vi "svx_Generate Excitation (DAQmx).vi"(0 "acquisition task":T1={"AI device settings"={"AI DAQmx TaskID"="", "response"=[{"AI physical channel"="Dev1/ai0", "AI channel settings"={"max value [V]"=10.0, "min value [V]"=-10.0, "terminal config"=10083, "DSA channel settings"={"coupling"=10045, "enable IEPE excitation"=FALSE, "IEPE current [mA]"=4.0}}}]}, "acquisition type"=enum."Finite", "measurement settings"={"AI sampling frequency"=51200.0, "AO sampling frequency"=51200.0, "AI block size"=0, "AO block Size"=0, "block duration [ms]"=100.0, "number of AI channels"=0, "device propagation delay [samples]"=0.0, "DUT propagation time [s]"=0.0}, "settling settings"={"settle time"=0.015599999576807022, "settle cycles"=5}, "integration settings"={"integration time"=0.015599999576807022, "integration cycles"=5}, "AO device settings"={"AO DAQmx taskID"="", "excitation"=[]}, "acquisition accounting"={"initial read size [samples]"=0, "read offset [samples]"=0, "read length [samples]"=0, "blocks to settle [samples]"=0, "min delay until transition [samples]"=0}, "frequency range"={"start frequency"=-1.0, "stop frequency"=-1.0}, "block type"=enum."Initialize", "source settings"={"signal type"=enum."Sine wave", "frequency"=0.0, "total amplitude"=0.0, "frequencies"=[1.0], "relative amplitudes"=[1.0], "offset"=1.0, "total amplitude list"=[1.0], "ramping rate"=0.0}, "chirp settings"={"amplitude"=0.0, "frequency range"={"start (Hz)"=20.0, "stop (Hz)"=20000.0, "frequency spacing"=enum."Logarithmic"}, "sampling info"={"Fs"=50000.0, "chirp duration [s]"=3.0}, "initial states"={"frequency [Hz]"=20.0, "phase [rad]"=0.0, "elapsed time [s]"=0.0}, "frequency slope"=0.0, "maximum harmonic"=0, "prefix len [samples]"={"integer"=0, "fractional"=0.0}}} {"chirp settings"."frequency slope" format="%.2f"; "chirp settings"."prefix len [samples]"."fractional" format="%.2p"; "chirp settings"."initial states"."elapsed time [s]" format="%.2f"; "chirp settings"."initial states"."phase [rad]" format="%.2f"; "chirp settings"."initial states"."frequency [Hz]" format="%.2f"; "chirp settings"."sampling info"."chirp duration [s]" format="%.2f"; "chirp settings"."sampling info"."Fs" format="%.2p"; "chirp settings"."frequency range"."stop (Hz)" format="%.2f"; "chirp settings"."frequency range"."start (Hz)" format="%.2f"; "chirp settings"."amplitude" format="%.2f"; "source settings"."total amplitude" format="%.2f"; "source settings"."relative amplitudes" format="%.2f"; "source settings"."frequencies" format="%.2f"; "source settings"."total amplitude list" format="%.2f"; "source settings"."ramping rate" format="%.4f"; "source settings"."offset" format="%.2f"; "source settings"."frequency" format="%.2f"; "frequency range"."stop frequency" format="%.2f"; "frequency range"."start frequency" format="%.2f"; "AO device settings"."excitation"."AO channel settings"."terminal config" items=["Default"=-1, "Differential"=10106, "Pseudodifferential"=12529]; "AI device settings"."response"."AI channel settings"."DSA channel settings"."IEPE current [mA]" min=0.0 max=20.0 format="%.1f"; "AI device settings"."response"."AI channel settings"."DSA channel settings"."coupling" items=["AC"=10045, "DC"=10050, "GND"=10066]; "AI device settings"."response"."AI channel settings"."min value [V]" format="%.2f"; "AI device settings"."response"."AI channel settings"."terminal config" items=["Default"=-1, "RSE"=10083, "NRSE"=10078, "Differential"=10106, "Pseudodifferential"=12529]; "AI device settings"."response"."AI channel settings"."max value [V]" format="%.2f"; "integration settings"."integration time" format="%.2p"; "settling settings"."settle time" format="%.2p"; "measurement settings"."DUT propagation time [s]" format="%.2f"; "measurement settings"."AO sampling frequency" format="%.2f"; "measurement settings"."AI sampling frequency" format="%.2f"}, 11 "error in (no error)":errorcluster, 12 "Iteration":i32) -> (4 "acquisition task out":T1={"AI device settings"={"AI DAQmx TaskID"="", "response"=[{"AI physical channel"="Dev1/ai0", "AI channel settings"={"max value [V]"=10.0, "min value [V]"=10.0, "terminal config"=-1, "DSA channel settings"={"coupling"=10045, "enable IEPE excitation"=FALSE, "IEPE current [mA]"=4.0}}}]}, "acquisition type"=enum."Finite", "measurement settings"={"AI sampling frequency"=0.0, "AO sampling frequency"=0.0, "AI block size"=0, "AO block Size"=0, "block duration [ms]"=100.0, "number of AI channels"=0, "device propagation delay [samples]"=0.0, "DUT propagation time [s]"=0.0}, "settling settings"={"settle time"=0.015599999576807022, "settle cycles"=5}, "integration settings"={"integration time"=0.015599999576807022, "integration cycles"=5}, "AO device settings"={"AO DAQmx taskID"="", "excitation"=[{"AO physical channel"="Dev1/ao0", "AO channel settings"={"maximum value (10 V)"=10.0, "minimum value (10 V)"=-10.0, "terminal config"=-1}}]}, "acquisition accounting"={"initial read size [samples]"=0, "read offset [samples]"=0, "read length [samples]"=0, "blocks to settle [samples]"=0, "min delay until transition [samples]"=0}, "frequency range"={"start frequency"=-1.0, "stop frequency"=-1.0}, "block type"=enum."Initialize", "source settings"={"signal type"=enum."Sine wave", "frequency"=0.0, "total amplitude"=0.0, "frequencies"=[1.0], "relative amplitudes"=[1.0], "offset"=1.0, "total amplitude list"=[1.0], "ramping rate"=0.0}, "chirp settings"={"amplitude"=0.0, "frequency range"={"start (Hz)"=20.0, "stop (Hz)"=20000.0, "frequency spacing"=enum."Logarithmic"}, "sampling info"={"Fs"=50000.0, "chirp duration [s]"=3.0}, "initial states"={"frequency [Hz]"=20.0, "phase [rad]"=0.0, "elapsed time [s]"=0.0}, "frequency slope"=0.0, "maximum harmonic"=0, "prefix len [samples]"={"integer"=0, "fractional"=0.0}}} {"chirp settings"."frequency slope" format="%.2f"; "chirp settings"."prefix len [samples]"."fractional" format="%.2p"; "chirp settings"."initial states"."elapsed time [s]" format="%.2f"; "chirp settings"."initial states"."phase [rad]" format="%.2f"; "chirp settings"."initial states"."frequency [Hz]" format="%.2f"; "chirp settings"."sampling info"."chirp duration [s]" format="%.2f"; "chirp settings"."sampling info"."Fs" format="%.2p"; "chirp settings"."frequency range"."stop (Hz)" format="%.2f"; "chirp settings"."frequency range"."start (Hz)" format="%.2f"; "chirp settings"."amplitude" format="%.2f"; "source settings"."total amplitude" format="%.2f"; "source settings"."relative amplitudes" format="%.2f"; "source settings"."frequencies" format="%.2f"; "source settings"."total amplitude list" format="%.2f"; "source settings"."ramping rate" format="%.4f"; "source settings"."offset" format="%.2f"; "source settings"."frequency" format="%.2f"; "frequency range"."stop frequency" format="%.2f"; "frequency range"."start frequency" format="%.2f"; "AO device settings"."excitation"."AO channel settings"."terminal config" items=["Default"=-1, "Differential"=10106, "Pseudodifferential"=12529]; "AI device settings"."response"."AI channel settings"."DSA channel settings"."IEPE current [mA]" min=0.0 max=20.0 format="%.1f"; "AI device settings"."response"."AI channel settings"."DSA channel settings"."coupling" items=["AC"=10045, "DC"=10050, "GND"=10066]; "AI device settings"."response"."AI channel settings"."min value [V]" format="%.2f"; "AI device settings"."response"."AI channel settings"."terminal config" items=["Default"=-1, "RSE"=10083, "NRSE"=10078, "Differential"=10106, "Pseudodifferential"=12529]; "AI device settings"."response"."AI channel settings"."max value [V]" format="%.2f"; "integration settings"."integration time" format="%.2p"; "settling settings"."settle time" format="%.2p"; "measurement settings"."DUT propagation time [s]" format="%.2f"; "measurement settings"."AO sampling frequency" format="%.2f"; "measurement settings"."AI sampling frequency" format="%.2f"}, 6 "waveform excitation":waveform(dbl)[](array[waveform]), 10 "end reached":bool, 15 "error out":errorcluster)   [LabVIEW 2017]
uses:
  <vilib>/addons/Sound and Vibration/Example Support/Audio/DAQmx/svx_Acquisition Task (DAQmx).ctl
  <vilib>/addons/_NISVFA/_Shared subVIs/Controls/svc_Channel Settings.ctl
  <vilib>/addons/_NISVFA/_Shared subVIs/Controls/svc_DSA Channel Settings.ctl
  <vilib>/addons/_NISVFA/_Generation/subVIs/sv_Chirp Settings.ctl
  <vilib>/addons/_NISVFA/_Generation/SoundVib_Generation.lvlib
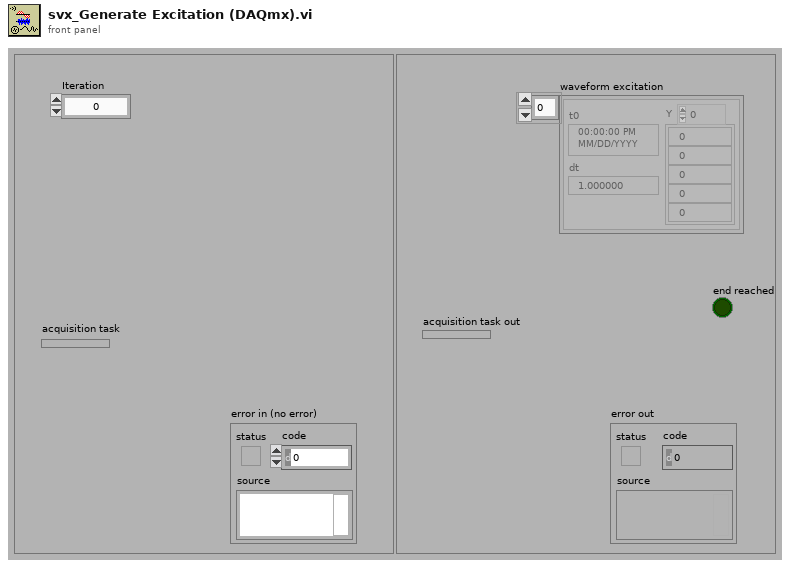
[diagram p1: front panel]
types:
  T1 = typedef "svx_Acquisition Task (DAQmx).ctl" = cluster{"AI device settings":cluster{"AI DAQmx TaskID":refnum<k21>, "response":cluster{"AI physical channel":tag, "AI channel settings":T2}[]}, "acquisition type":enum16{"Finite", "Averaged", "Settled", "Amplitude Sweep", "Stepped Frequency Sweep", "Continuous Frequency Sweep"}, "measurement settings":cluster{"AI sampling frequency":dbl, "AO sampling frequency":dbl, "AI block size":i32, "AO block Size":i32, "block duration [ms]":dbl, "number of AI channels":i32, "device propagation delay [samples]":dbl, "DUT propagation time [s]":dbl}, "settling settings":cluster{"settle time":dbl, "settle cycles":i32}, "integration settings":cluster{"integration time":dbl, "integration cycles":i32}, "AO device settings":cluster{"AO DAQmx taskID":refnum<k21>, "excitation":cluster{"AO physical channel":tag, "AO channel settings":cluster{"maximum value (10 V)":dbl, "minimum value (10 V)":dbl, "terminal config":i32}}[]}, "acquisition accounting":cluster{"initial read size [samples]":i32, "read offset [samples]":i32, "read length [samples]":i32, "blocks to settle [samples]":i32, "min delay until transition [samples]":i32}, "frequency range":cluster{"start frequency":dbl, "stop frequency":dbl}, "block type":enum16{"Initialize", "Settle", "Integrate"}, "source settings":cluster{"signal type":enum16{"Sine wave", "Dual tone (IMD)", "Multitone", "Chirp", "Frequency flat chirp", "Uniform white noise", "Gaussian white noise", "Pink noise", "PRN", "Continuous swept-sine"}, "frequency":dbl, "total amplitude":dbl, "frequencies":dbl[], "relative amplitudes":dbl[], "offset":dbl, "total amplitude list":dbl[], "ramping rate":dbl}, "chirp settings":T4}
  T2 = typedef "svc_Channel Settings.ctl" = cluster{"max value [V]":dbl, "min value [V]":dbl, "terminal config":i32, "DSA channel settings":T3}
  T3 = typedef "svc_DSA Channel Settings.ctl" = cluster{"coupling":i32, "enable IEPE excitation":bool, "IEPE current [mA]":dbl}
  T4 = typedef "SoundVib_Generation.lvlib/sv_Chirp Settings.ctl" = cluster{"amplitude":dbl, "frequency range":cluster{"start (Hz)":dbl, "stop (Hz)":dbl, "frequency spacing":enum16{"Linear", "Logarithmic"}}, "sampling info":cluster{"Fs":dbl, "chirp duration [s]":dbl}, "initial states":cluster{"frequency [Hz]":dbl, "phase [rad]":dbl, "elapsed time [s]":dbl}, "frequency slope":dbl, "maximum harmonic":i32, "prefix len [samples]":cluster{"integer":u32, "fractional":dbl}}
  T5 = cluster{"amplitude":dbl, "offset":dbl, "tf (ignored)":dbl}
  T6 = cluster{"frequency":dbl, "amplitude":dbl, "offset":dbl, "phase":dbl, "tf (ignored)":dbl}
  T7 = cluster{"frequencies":dbl[], "relative amplitudes":dbl[], "phases":dbl[], "total amplitude":dbl, "offset":dbl, "tf (ignored)":dbl}
  T8 = enum16{"Reset", "Continue from previous", "Continue from state", "Zero from previous", "Zero from state"}
  T9 = enum16{"Sine wave", "Dual tone (IMD)", "Multitone", "Chirp", "Frequency flat chirp", "Uniform white noise", "Gaussian white noise", "Pink noise", "PRN", "Continuous swept-sine"}
  T10 = enum16{"Finite", "Averaged", "Settled", "Amplitude Sweep", "Stepped Frequency Sweep", "Continuous Frequency Sweep"}
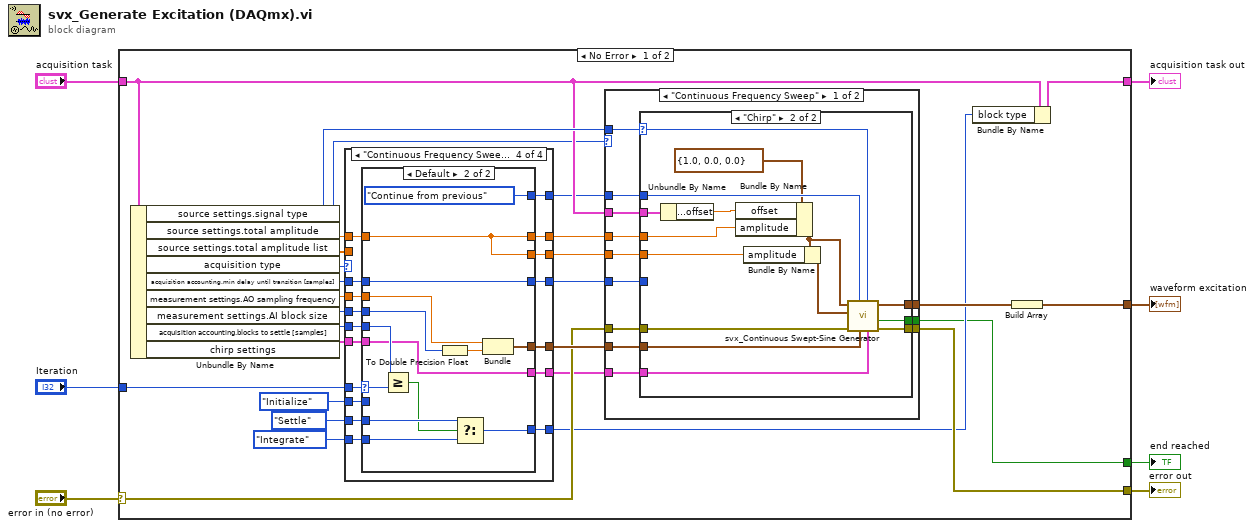
[diagram p0: block diagram]
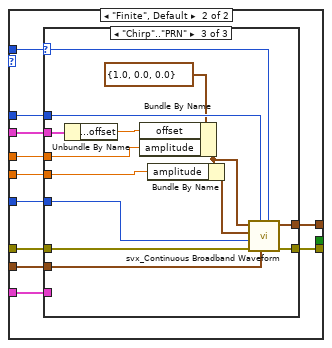
[diagram p3: hidden frame]
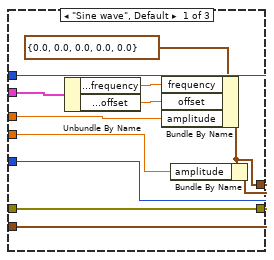
[diagram p4: hidden frame]
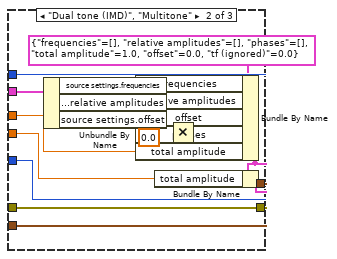
[diagram p5: hidden frame]
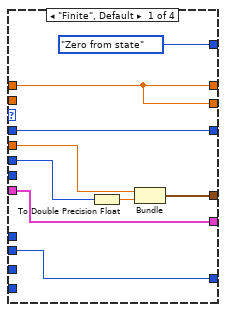
[diagram p6: hidden frame]
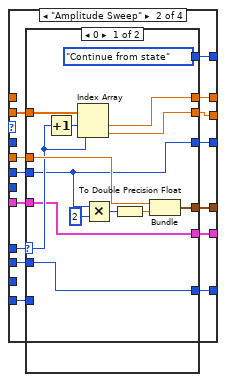
[diagram p7: hidden frame]
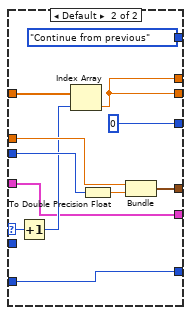
[diagram p8: hidden frame]
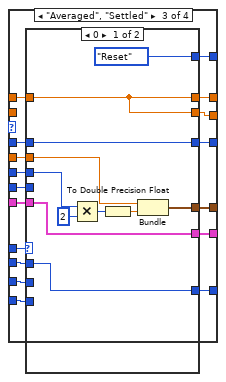
[diagram p9: hidden frame]
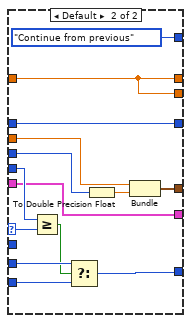
[diagram p10: hidden frame]
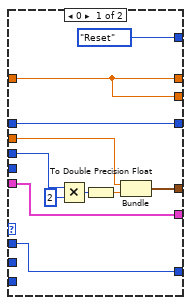
[diagram p11: hidden frame]
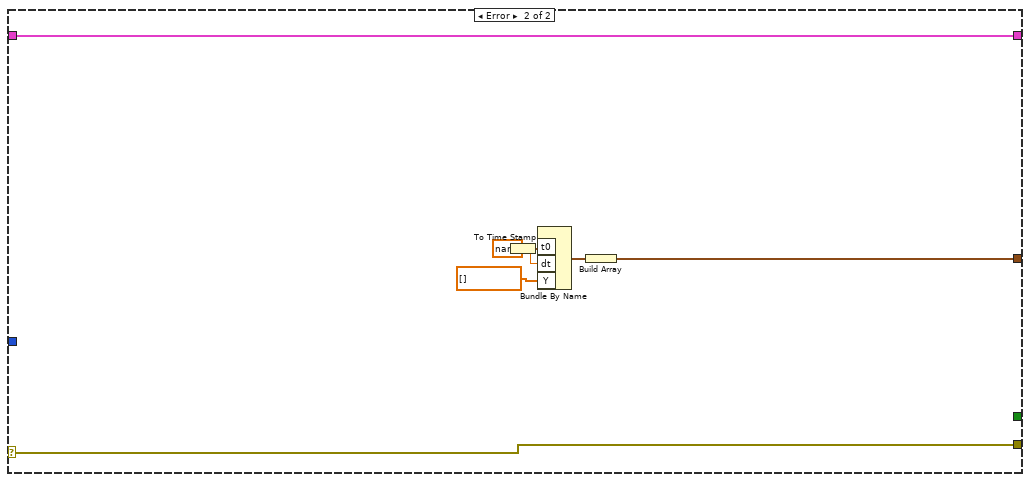
[diagram p12: hidden frame]
diagram:
  n1 = case shown="No Error" "error in (no error)" {
    selector: "error in (no error)" -> [w14 w260]
    tunnel: [w34 w256] -> w7
    tunnel: [w32 w260] -> w6
    tunnel: "acquisition task" -> [w18 w255]
    tunnel: [w30 w255] -> w1
    tunnel: "Iteration" -> [w22 _]
    tunnel: [w8 _] -> w2
    frame No Error {
      n2 = Unbundle By Name(w18) -> ("source settings.signal type"=w31:T9, "source settings.total amplitude"=w19:dbl, "source settings.total amplitude list"=w23:dbl[], "acquisition type"=w9:T10, "acquisition accounting.min delay until transition [samples]"=w25:i32, "measurement settings.AO sampling frequency"=w24:dbl, "measurement settings.AI block size"=w21:i32, "acquisition accounting.blocks to settle [samples]"=w26:i32, "chirp settings"=w11:T4)
      n3 = case shown="\"Continuous Frequency Sweep\"" w9 {
        tunnel: [w129 w140 w179 w221] -> w20
        tunnel: w21 -> [w128 w139 w182 w224]
        tunnel: [T8."Zero from state" ("generation control") w143 w180 w222] -> w16
        tunnel: [w124 w142 w177 w219] -> w15
        tunnel: w22 -> [_ w141 w186 w228]
        tunnel: enum16{"Initialize", "Settle", "Integrate"}."Initialize" ("block type") -> [w125 w137 w178 w220]
        tunnel: enum16{"Initialize", "Settle", "Integrate"}."Settle" ("block type") -> [_ _ w184 w226]
        tunnel: enum16{"Initialize", "Settle", "Integrate"}."Integrate" ("block type") -> [_ w136 w183 w225]
        tunnel: [w125 w138 w185 w227] -> w13
        tunnel: w26 -> [_ _ w181 w223]
        tunnel: w25 -> [w124 _ w174 w216]
        tunnel: w24 -> [w123 w135 w176 w218]
        tunnel: w19 -> [w122 _ w175 w217]
        tunnel: w23 -> [_ w134 _ _]
        tunnel: [w122 w132 w173 w215] -> w17
        tunnel: [w122 w133 w172 w214] -> w12
        tunnel: w11 -> [w121 w130 w171 w213]
        tunnel: [w121 w131 w170 w212] -> w10
        frame "Finite", Default {
          n4 = To Double Precision Float(number=w128) -> (double precision float=w127:dbl)
          n5 = Bundle("AO sampling frequency"=w123, w127) -> (w129:cluster{"AO sampling frequency":dbl, dbl})  [unwired: 1 in]
        }
        frame "Amplitude Sweep" {
          n6 = case shown="0" w141 {
            selector: w141 -> [w148 w163]
            tunnel: [T8."Continue from state" ("generation control") T8."Continue from previous" ("generation control")] -> w143
            tunnel: [w147 0] -> w142
            tunnel: [w155 w167] -> w140
            tunnel: w139 -> [w147 w166]
            tunnel: w135 -> [w152 w165]
            tunnel: w134 -> [w151 w161]
            tunnel: [w146 w160] -> w138
            tunnel: w137 -> [w146 _]
            tunnel: w136 -> [_ w160]
            tunnel: [w145 w159] -> w133
            tunnel: [w149 w159] -> w132
            tunnel: [w144 w158] -> w131
            tunnel: w130 -> [w144 w158]
            frame 0 {
              n7 = Increment(x=w148) -> (x+1=w150:i32)
              n8 = Index Array(array=w151, index #1=w150, index #2=w148) -> (element #1=w149:dbl, element #2=w145:dbl)
              n9 = Multiply(x=w147, y=2) -> (x*y=w154:i32)
              n10 = To Double Precision Float(number=w154) -> (double precision float=w156:dbl)
              n11 = Bundle("AO sampling frequency"=w152, w156) -> (w155:cluster{"AO sampling frequency":dbl, dbl})  [unwired: 1 in]
            }
            frame Default {
              n12 = Increment(x=w163) -> (x+1=w162:i32)
              n13 = Index Array(array=w161, index=w162) -> (element=w159:dbl)
              n14 = To Double Precision Float(number=w166) -> (double precision float=w168:dbl)
              n15 = Bundle("AO sampling frequency"=w165, w168) -> (w167:cluster{"AO sampling frequency":dbl, dbl})  [unwired: 1 in]
            }
          }
        }
        frame "Averaged", "Settled" {
          n16 = case shown="0" w186 {
            selector: w186 -> [_ w204]
            tunnel: [w196 w210] -> w179
            tunnel: w182 -> [w191 w209]
            tunnel: w176 -> [w193 w208]
            tunnel: [w192 w202] -> w185
            tunnel: w178 -> [w192 _]
            tunnel: w183 -> [_ w207]
            tunnel: w184 -> [_ w206]
            tunnel: w181 -> [_ w205]
            tunnel: [T8."Reset" ("generation control") T8."Continue from previous" ("generation control")] -> w180
            tunnel: [w189 w199] -> w177
            tunnel: w175 -> [w188 w200]
            tunnel: w174 -> [w189 w199]
            tunnel: [w188 w200] -> w173
            tunnel: [w188 w200] -> w172
            tunnel: w171 -> [w187 w198]
            tunnel: [w187 w198] -> w170
            frame 0 {
              n17 = Multiply(x=w191, y=2) -> (x*y=w195:i32)
              n18 = To Double Precision Float(number=w195) -> (double precision float=w197:dbl)
              n19 = Bundle("AO sampling frequency"=w193, w197) -> (w196:cluster{"AO sampling frequency":dbl, dbl})  [unwired: 1 in]
            }
            frame Default {
              n20 = Greater Or Equal?(x=w205, y=w204) -> (x >= y?=w203:bool)
              n21 = Select(t=w206, s=w203, f=w207) -> (s? t:f=w202:enum16{"Initialize", "Settle", "Integrate"})
              n22 = To Double Precision Float(number=w209) -> (double precision float=w211:dbl)
              n23 = Bundle("AO sampling frequency"=w208, w211) -> (w210:cluster{"AO sampling frequency":dbl, dbl})  [unwired: 1 in]
            }
          }
        }
        frame "Continuous Frequency Sweep" {
          n24 = case shown="Default" w228 {
            selector: w228 -> [_ w240]
            tunnel: [w238 w252] -> w221
            tunnel: w224 -> [w233 w251]
            tunnel: w218 -> [w235 w250]
            tunnel: [w234 w245] -> w227
            tunnel: w220 -> [w234 _]
            tunnel: w225 -> [_ w249]
            tunnel: w226 -> [_ w248]
            tunnel: w223 -> [_ w247]
            tunnel: [T8."Reset" ("generation control") T8."Continue from previous" ("generation control")] -> w222
            tunnel: [w231 w242] -> w219
            tunnel: w217 -> [w230 w243]
            tunnel: w216 -> [w231 w242]
            tunnel: [w230 w243] -> w215
            tunnel: [w230 w243] -> w214
            tunnel: w213 -> [w229 w241]
            tunnel: [w229 w241] -> w212
            frame 0 {
              n25 = Multiply(x=w233, y=2) -> (x*y=w237:i32)
              n26 = To Double Precision Float(number=w237) -> (double precision float=w239:dbl)
              n27 = Bundle("AO sampling frequency"=w235, w239) -> (w238:cluster{"AO sampling frequency":dbl, dbl})  [unwired: 1 in]
            }
            frame Default {
              n28 = Greater Or Equal?(x=w247, y=w240) -> (x >= y?=w246:bool)
              n29 = To Double Precision Float(number=w251) -> (double precision float=w253:dbl)
              n30 = Select(t=w248, s=w246, f=w249) -> (s? t:f=w245:enum16{"Initialize", "Settle", "Integrate"})
              n31 = Bundle("AO sampling frequency"=w250, w253) -> (w252:cluster{"AO sampling frequency":dbl, dbl})  [unwired: 1 in]
            }
          }
        }
      }
      n32 = case shown="\"Continuous Frequency Sweep\"" w9 {
        tunnel: [w46 w75] -> w33
        tunnel: [w45 w74] -> w32
        tunnel: w31 -> [w44 w73]
        tunnel: w20 -> [w43 w72]
        tunnel: w18 -> [w42 w71]
        tunnel: w17 -> [w41 w70]
        tunnel: w16 -> [w40 w69]
        tunnel: w15 -> [w39 w68]
        tunnel: w14 -> [w38 w67]
        tunnel: w12 -> [w37 w66]
        tunnel: w10 -> [w36 w65]
        tunnel: [w35 _] -> w8
        frame "Continuous Frequency Sweep" {
          n33 = case shown="\"Chirp\"" w44 {
            selector: w44 -> [_ w52]
            tunnel: [w49 w62] -> w46
            tunnel: w38 -> [w48 w64]
            tunnel: [w47 w63] -> w45
            tunnel: w43 -> [_ w57]
            tunnel: w42 -> [_ w61]
            tunnel: w41 -> [_ w60]
            tunnel: w40 -> [_ w58]
            tunnel: w39 -> [_ _]
            tunnel: w37 -> [_ w59]
            tunnel: w36 -> [_ w51]
            tunnel: [_ w50] -> w35
            frame "Sine wave", Default {
              n34 = call <vilib>:"svx_Continuous Sine Waveform.vi"("error in"=w48) -> ("error out"=w47:errorcluster, "signal out"=w49:waveform(dbl))  [unwired: 7 in, 2 out]
            }
            frame "Chirp" {
              n35 = Unbundle By Name(w61) -> ("source settings.offset"=w56:dbl)
              n36 = Bundle By Name(cluster=T5 {"amplitude"=1.0, "offset"=0.0, "tf (ignored)"=0.0} ("desired waveform state"), "offset"=w56, "amplitude"=w60) -> (w54:T5)
              n37 = Bundle By Name(cluster=w54, "amplitude"=w59) -> (w53:T5)
              n38 = call <vilib>:"svx_Continuous Swept-Sine Generator.vi"("chirp settings"=w51, "signal type"=w52, "sampling info"=w57, "generation control"=w58, "error in"=w64, "initial waveform state"=w53, "desired waveform state"=w54) -> ("error out"=w63:errorcluster, "end reached?"=w50:bool, "signal out"=w62:waveform(dbl))  [unwired: 1 in, 1 out]
            }
          }
        }
        frame "Finite", Default {
          n39 = case shown="\"Chirp\"..\"PRN\"" w73 {
            selector: w73 -> [_ _ w107]
            tunnel: [w89 w106 w118] -> w75
            tunnel: w67 -> [w88 w105 w120]
            tunnel: [w87 w104 w119] -> w74
            tunnel: w72 -> [w86 w103 w113]
            tunnel: w71 -> [w85 w90 w117]
            tunnel: w70 -> [w78 w102 w116]
            tunnel: w69 -> [w82 w101 w114]
            tunnel: w68 -> [w81 w100 w108]
            tunnel: w66 -> [w80 w93 w115]
            tunnel: w65 -> [_ _ _]
            frame "Sine wave", Default {
              n40 = Unbundle By Name(w85) -> ("source settings.frequency"=w84:dbl, "source settings.offset"=w83:dbl)
              n41 = Bundle By Name(cluster=T6 {"frequency"=0.0, "amplitude"=0.0, "offset"=0.0, "phase"=0.0, "tf (ignored)"=0.0} ("desired waveform state"), "frequency"=w84, "offset"=w83, "amplitude"=w78) -> (w77:T6)
              n42 = Bundle By Name(cluster=w77, "amplitude"=w80) -> (w76:T6)
              n43 = call <vilib>:"svx_Continuous Sine Waveform.vi"("sampling info"=w86, "generation control"=w82, "error in"=w88, "delay until transition (0 samples)"=w81, "current waveform state"=w76, "desired waveform state"=w77) -> ("error out"=w87:errorcluster, "signal out"=w89:waveform(dbl))  [unwired: 2 in, 2 out]
            }
            frame "Dual tone (IMD)", "Multitone" {
              n44 = Unbundle By Name(w90) -> ("source settings.frequencies"=w98:dbl[], "source settings.relative amplitudes"=w96:dbl[], "source settings.offset"=w97:dbl)
              n45 = Multiply(x=w96, y=0.0 ("offset")) -> (x*y=w95:dbl[])
              n46 = Bundle By Name(cluster=T7 {"frequencies"=[], "relative amplitudes"=[], "phases"=[], "total amplitude"=1.0, "offset"=0.0, "tf (ignored)"=0.0} ("desired waveform state"), "frequencies"=w98, "relative amplitudes"=w96, "offset"=w97, "phases"=w95, "total amplitude"=w102) -> (w92:T7)
              n47 = Bundle By Name(cluster=w92, "total amplitude"=w93) -> (w91:T7)
              n48 = call <vilib>:"svx_Continuous Multitone Waveform.vi"("sampling info"=w103, "generation control"=w101, "error in"=w105, "delay until transition (0 samples)"=w100, "initial waveform state"=w91, "desired waveform state"=w92) -> ("error out"=w104:errorcluster, "signal out"=w106:waveform(dbl))  [unwired: 2 in, 2 out]
            }
            frame "Chirp".."PRN" {
              n49 = Unbundle By Name(w117) -> ("source settings.offset"=w112:dbl)
              n50 = Bundle By Name(cluster=T5 {"amplitude"=1.0, "offset"=0.0, "tf (ignored)"=0.0} ("desired waveform state"), "offset"=w112, "amplitude"=w116) -> (w110:T5)
              n51 = Bundle By Name(cluster=w110, "amplitude"=w115) -> (w109:T5)
              n52 = call <vilib>:"svx_Continuous Broadband Waveform.vi"("signal type"=w107, "sampling info"=w113, "generation control"=w114, "error in"=w120, "delay until transition (0 samples)"=w108, "initial waveform state"=w109, "desired waveform state"=w110) -> ("error out"=w119:errorcluster, "signal out"=w118:waveform(dbl))  [unwired: 1 in, 2 out]
            }
          }
        }
      }
      n53 = Bundle By Name(cluster=w18, "block type"=w13) -> (w30:T1)
      n54 = Build Array(w33) -> (w34:waveform(dbl)[])
    }
    frame Error {
      w258 = nan ("t0")
      n55 = To Time Stamp(1:w258) -> (0:w254:timestamp)
      n56 = Bundle By Name("t0"=w254, "dt"=w258, "Y"=dbl[] []) -> (w257:waveform(dbl))  [unwired: 1 in]
      n57 = Build Array(w257) -> (w256:waveform(dbl)[])
    }
  }
  "error out" <- w6
  "waveform excitation" <- w7
  "end reached" <- w2
  "acquisition task out" <- w1
